vi "step3 TestAndSolveMiddleLayerEdge.vi"(11 "cube in":T1) -> (3 "cube out":T1)   [LabVIEW 2011]
uses:
  Typedef/cube.ctl
  Typedef/face.ctl
  Typedef/cube rotate direction.ctl
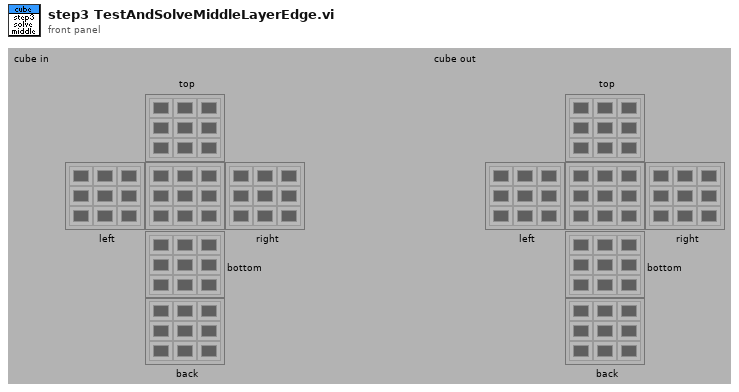
[diagram p1: front panel]
types:
  T1 = typedef "cube.ctl" = cluster{"top":T2, "left":T2, "right":T2, "bottom":T2, "back":T2, "front":T2}
  T2 = typedef "face.ctl" = u32[][]
  T3 = typedef "cube rotate direction.ctl" = enum16{"up", "down", "left", "right"}
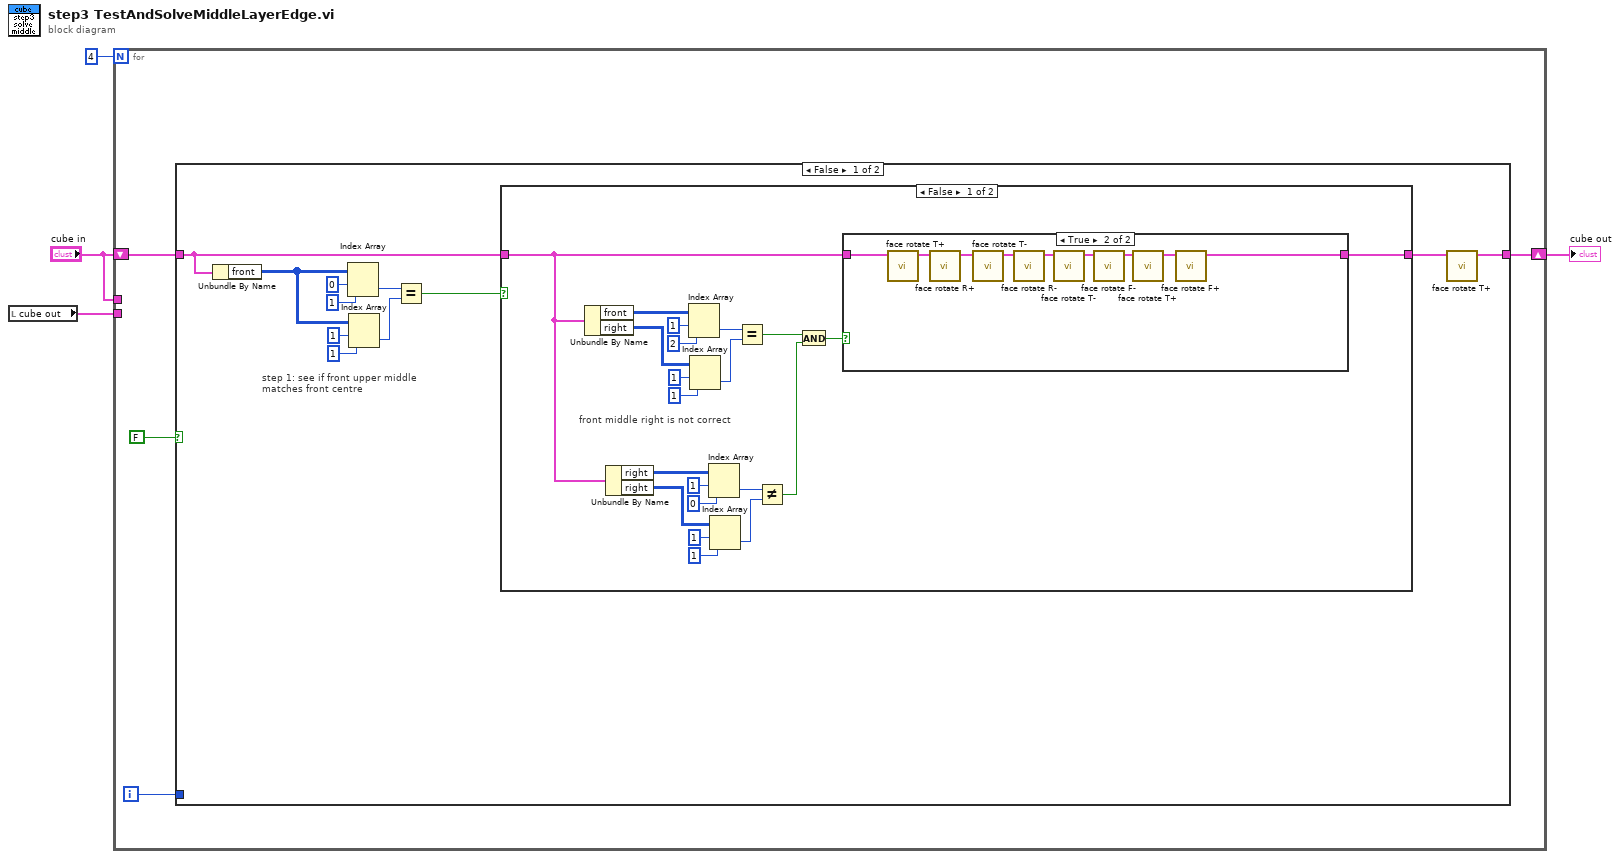
[diagram p0: block diagram]
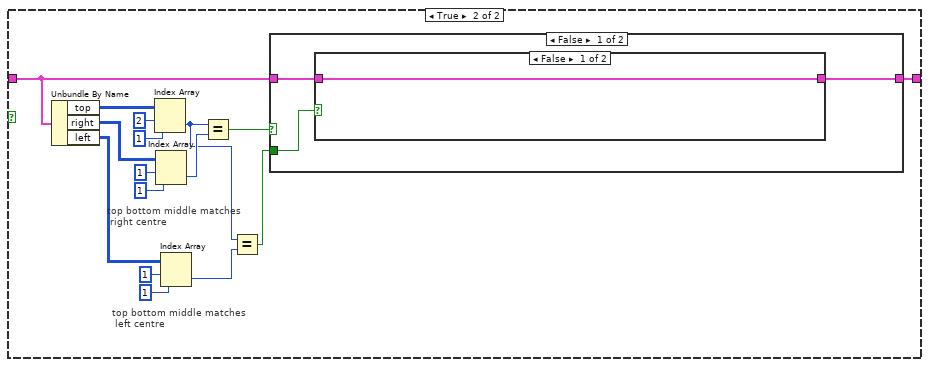
[diagram p3: hidden frame]
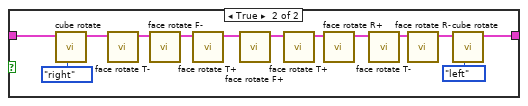
[diagram p4: hidden frame]
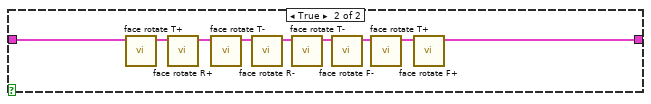
[diagram p5: hidden frame]
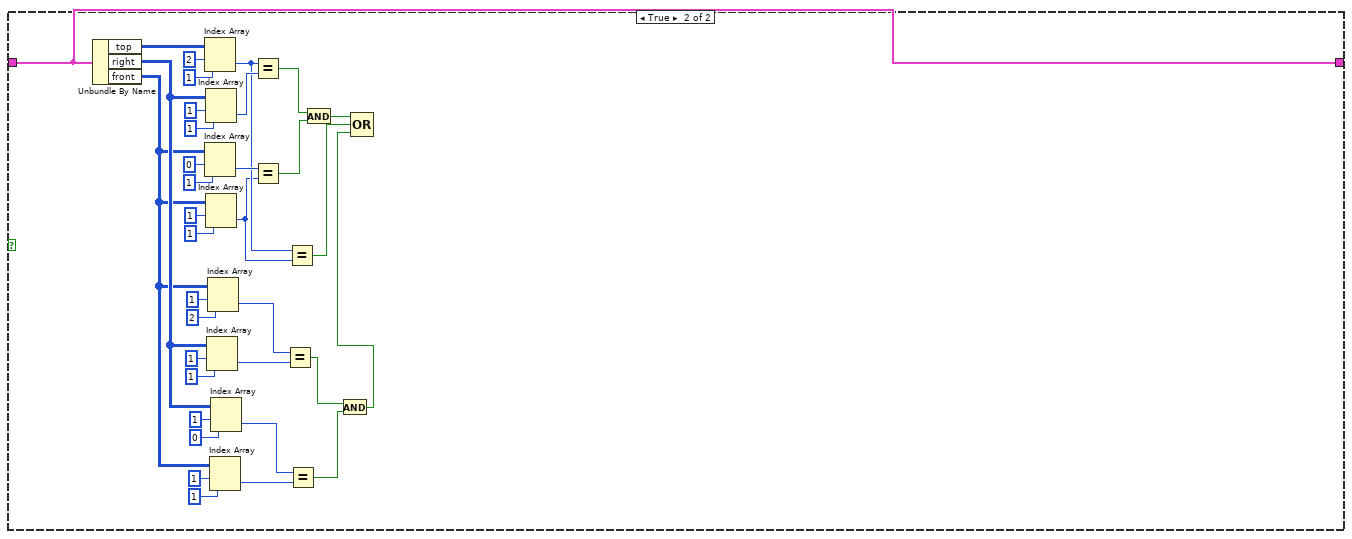
[diagram p6: hidden frame]
diagram:
  n1 = local read "cube out"() -> (w2:T1)
  n2 = for {
    N: 4 -> [_]
    shift-right: [w6] -> w1
    shift-left: "cube in" -> [w8]
    tunnel: "cube in" -> [_]
    tunnel: w2 -> [_]
    i -> [w5]
    n3 = case shown="False" FALSE {
      tunnel: w8 -> [w10 w93]
      tunnel: [w12 w93] -> w6
      tunnel: w5 -> [_ _]
      frame False {
        # "step 1: see if front upper middle \nmatches front centre"
        n4 = Unbundle By Name(w10) -> ("front"=w13:T2)
        n5 = Index Array(array=w13, index (row)=0, index (col)=1 ("disabled index (col)")) -> (element=w19:u32)
        n6 = Index Array(array=w13, index (row)=1, index (col)=1 ("disabled index (col)")) -> (element=w18:u32)
        n7 = Equal?(x=w19, y=w18) -> (x = y?=w11:bool)
        n8 = case shown="False" w11 {
          tunnel: w10 -> [w22 w55]
          tunnel: [w21 w51] -> w9
          frame False {
            # "front middle right is not correct"
            n9 = Unbundle By Name(w22) -> ("front"=w33:T2, "right"=w34:T2)
            n10 = Unbundle By Name(w22) -> ("right"=w31:T2, "right"=w30:T2)
            n11 = Index Array(array=w33, index (row)=1, index (col)=2 ("disabled index (col)")) -> (element=w40:u32)
            n12 = Index Array(array=w34, index (row)=1, index (col)=1 ("disabled index (col)")) -> (element=w39:u32)
            n13 = Index Array(array=w31, index (row)=1, index (col)=0 ("disabled index (col)")) -> (element=w24:u32)
            n14 = Index Array(array=w30, index (row)=1, index (col)=1 ("disabled index (col)")) -> (element=w25:u32)
            n15 = Equal?(x=w40, y=w39) -> (x = y?=w32:bool)
            n16 = Not Equal?(x=w24, y=w25) -> (x != y?=w23:bool)
            n17 = And(x=w32, y=w23) -> (x .and. y?=w20:bool)
            n18 = case shown="True" w20 {
              tunnel: w22 -> [w41 w43]
              tunnel: [w41 w42] -> w21
              frame False {
              }
              frame True {
                n19 = call "face rotate T+.vi"("cube in"=w43) -> ("cube out"=w44:T1)  [unwired: 9 in, 1 out]
                n20 = call "face rotate R+.vi"("cube in"=w44) -> ("cube out"=w45:T1)  [unwired: 9 in, 1 out]
                n21 = call "face rotate T-.vi"("cube in"=w45) -> ("cube out"=w46:T1)  [unwired: 9 in, 1 out]
                n22 = call "face rotate R-.vi"("cube in"=w46) -> ("cube out"=w47:T1)  [unwired: 9 in, 1 out]
                n23 = call "face rotate T-.vi"("cube in"=w47) -> ("cube out"=w48:T1)  [unwired: 9 in, 1 out]
                n24 = call "face rotate F-.vi"("cube in"=w48) -> ("cube out"=w49:T1)  [unwired: 9 in, 1 out]
                n25 = call "face rotate T+.vi"("cube in"=w49) -> ("cube out"=w50:T1)  [unwired: 9 in, 1 out]
                n26 = call "face rotate F+.vi"("cube in"=w50) -> ("cube out"=w42:T1)  [unwired: 9 in, 1 out]
              }
            }
          }
          frame True {
            # "top bottom middle matches\n left centre"
            # "top bottom middle matches\n right centre"
            n27 = Unbundle By Name(w55) -> ("top"=w65:T2, "right"=w66:T2, "left"=w56:T2)
            n28 = Index Array(array=w65, index (row)=2, index (col)=1 ("disabled index (col)")) -> (element=w54:u32)
            n29 = Index Array(array=w66, index (row)=1, index (col)=1 ("disabled index (col)")) -> (element=w64:u32)
            n30 = Index Array(array=w56, index (row)=1, index (col)=1 ("disabled index (col)")) -> (element=w53:u32)
            n31 = Equal?(x=w54, y=w64) -> (x = y?=w59:bool)
            n32 = Equal?(x=w54, y=w53) -> (x = y?=w52:bool)
            n33 = case shown="False" w59 {
              tunnel: w55 -> [w69 w85]
              tunnel: [w68 w84] -> w51
              tunnel: w52 -> [w67 _]
              frame False {
                n34 = case shown="False" w67 {
                  tunnel: w69 -> [w70 w75]
                  tunnel: [w70 w71] -> w68
                  frame False {
                  }
                  frame True {
                    n35 = call "cube rotate.vi"("cube rotation direction"=cube_rotate_direction."right", "cube in"=w75) -> ("cube out"=w74:T1)  [unwired: 8 in, 1 out]
                    n36 = call "face rotate T-.vi"("cube in"=w74) -> ("cube out"=w77:T1)  [unwired: 9 in, 1 out]
                    n37 = call "face rotate F-.vi"("cube in"=w77) -> ("cube out"=w78:T1)  [unwired: 9 in, 1 out]
                    n38 = call "face rotate T+.vi"("cube in"=w78) -> ("cube out"=w79:T1)  [unwired: 9 in, 1 out]
                    n39 = call "face rotate F+.vi"("cube in"=w79) -> ("cube out"=w80:T1)  [unwired: 9 in, 1 out]
                    n40 = call "face rotate T+.vi"("cube in"=w80) -> ("cube out"=w81:T1)  [unwired: 9 in, 1 out]
                    n41 = call "face rotate R+.vi"("cube in"=w81) -> ("cube out"=w82:T1)  [unwired: 9 in, 1 out]
                    n42 = call "face rotate T-.vi"("cube in"=w82) -> ("cube out"=w83:T1)  [unwired: 9 in, 1 out]
                    n43 = call "face rotate R-.vi"("cube in"=w83) -> ("cube out"=w72:T1)  [unwired: 9 in, 1 out]
                    n44 = call "cube rotate.vi"("cube rotation direction"=cube_rotate_direction."left", "cube in"=w72) -> ("cube out"=w71:T1)  [unwired: 8 in, 1 out]
                  }
                }
              }
              frame True {
                n45 = call "face rotate T+.vi"("cube in"=w85) -> ("cube out"=w86:T1)  [unwired: 9 in, 1 out]
                n46 = call "face rotate R+.vi"("cube in"=w86) -> ("cube out"=w87:T1)  [unwired: 9 in, 1 out]
                n47 = call "face rotate T-.vi"("cube in"=w87) -> ("cube out"=w88:T1)  [unwired: 9 in, 1 out]
                n48 = call "face rotate R-.vi"("cube in"=w88) -> ("cube out"=w89:T1)  [unwired: 9 in, 1 out]
                n49 = call "face rotate T-.vi"("cube in"=w89) -> ("cube out"=w90:T1)  [unwired: 9 in, 1 out]
                n50 = call "face rotate F-.vi"("cube in"=w90) -> ("cube out"=w91:T1)  [unwired: 9 in, 1 out]
                n51 = call "face rotate T+.vi"("cube in"=w91) -> ("cube out"=w92:T1)  [unwired: 9 in, 1 out]
                n52 = call "face rotate F+.vi"("cube in"=w92) -> ("cube out"=w84:T1)  [unwired: 9 in, 1 out]
              }
            }
          }
        }
        n53 = call "face rotate T+.vi"("cube in"=w9) -> ("cube out"=w12:T1)  [unwired: 9 in, 1 out]
      }
      frame True {
        n54 = Unbundle By Name(w93) -> ("top"=w127:T2, "right"=w98:T2, "front"=w97:T2)
        n55 = Index Array(array=w127, index (row)=2, index (col)=1 ("disabled index (col)")) -> (element=w113:u32)
        n56 = Index Array(array=w97, index (row)=0, index (col)=1 ("disabled index (col)")) -> (element=w122:u32)
        n57 = Index Array(array=w98, index (row)=1, index (col)=1 ("disabled index (col)")) -> (element=w114:u32)
        n58 = Index Array(array=w97, index (row)=1, index (col)=1 ("disabled index (col)")) -> (element=w112:u32)
        n59 = Index Array(array=w98, index (row)=1, index (col)=1 ("disabled index (col)")) -> (element=w105:u32)
        n60 = Index Array(array=w97, index (row)=1, index (col)=2 ("disabled index (col)")) -> (element=w106:u32)
        n61 = Index Array(array=w97, index (row)=1, index (col)=1 ("disabled index (col)")) -> (element=w104:u32)
        n62 = Index Array(array=w98, index (row)=1, index (col)=0 ("disabled index (col)")) -> (element=w103:u32)
        n63 = Equal?(x=w113, y=w114) -> (x = y?=w117:bool)
        n64 = Equal?(x=w122, y=w112) -> (x = y?=w116:bool)
        n65 = Equal?(x=w106, y=w105) -> (x = y?=w96:bool)
        n66 = Equal?(x=w113, y=w112) -> (x = y?=w111:bool)
        n67 = Equal?(x=w103, y=w104) -> (x = y?=w95:bool)
        n68 = And(x=w117, y=w116) -> (x .and. y?=w115:bool)
        n69 = And(x=w96, y=w95) -> (x .and. y?=w94:bool)
        n70 = Compound Arithmetic op=OR(w115, w111, w94) -> ()  [unwired: 1 out]
      }
    }
  }
  "cube out" <- w1
